vi "Draw Note on Staff.vi"(7 "Landmark C's":bool, 10 "Note Number":i16, 11 "Clef":T1) -> (3 "picture out":picture)   [LabVIEW 2014]
uses:
  Type Defs/Clef.ctl
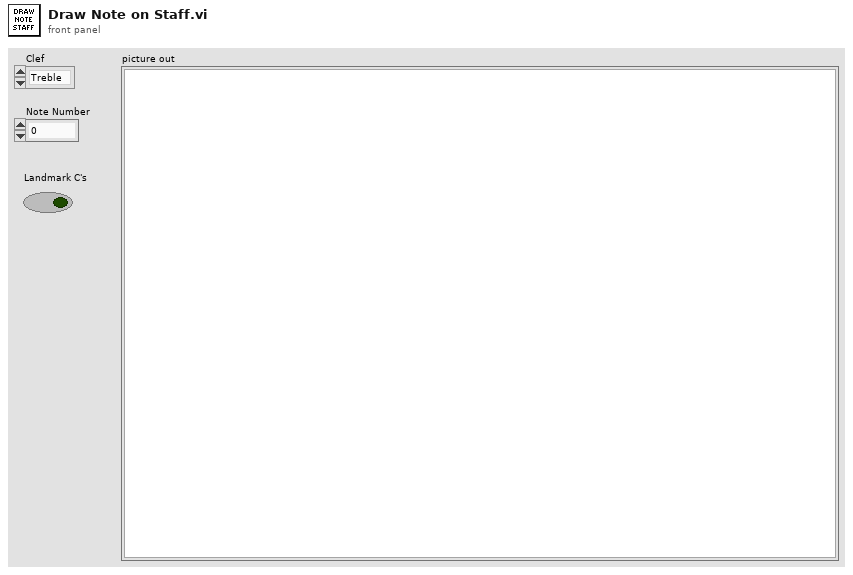
[diagram p1: front panel]
types:
  T1 = typedef "Clef.ctl" = enum16{"Treble", "Bass"}
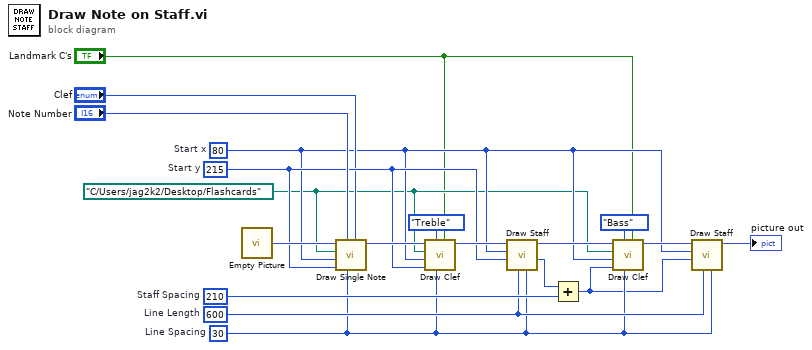
[diagram p0: block diagram]
diagram:
  w2 = path "C:/Users/jag2k2/Desktop/Flashcards" ("Picture Path")
  w12 = i16 215  # Start y
  w7 = i16 80  # Start x
  w19 = i16 210  # Staff Spacing
  w6 = i16 30  # Line Spacing
  w17 = i16 600  # Line Length
  n1 = call "Empty Picture"() -> ("empty picture"=w16:picture)
  n2 = call "Draw Single Note.vi"("Clef"="Clef", "Line Spacing"=w6, "Note Number"="Note Number", "Start y"=w12, "Start x"=w7, "Picture Path"=w2, "Picture In"=w16) -> ("Picture Out"=w14:picture)  [unwired: 4 in]
  n3 = call "Draw Clef.vi"("Landmark C's"="Landmark C's", "Line Spacing"=w6, "Clef"=Clef."Treble", "Start y"=w12, "Start x"=w7, "Picture Path"=w2, "Picture In"=w14) -> ("Picture Out"=w13:picture)  [unwired: 4 in]
  n4 = call "Draw Staff.vi"("Line Spacing"=w6, "Line Length"=w17, "Start y"=w12, "Start x"=w7, "picture in"=w13) -> ("End y"=w18:i16, "picture out"=w9:picture)  [unwired: 5 in]
  n5 = Add(x=w18, y=w19) -> (x+y=w5:i16)
  n6 = call "Draw Clef.vi"("Landmark C's"="Landmark C's", "Line Spacing"=w6, "Clef"=Clef."Bass", "Start y"=w5, "Start x"=w7, "Picture Path"=w2, "Picture In"=w9) -> ("Picture Out"=w8:picture)  [unwired: 4 in]
  n7 = call "Draw Staff.vi"("Line Spacing"=w6, "Line Length"=w17, "Start y"=w5, "Start x"=w7, "picture in"=w8) -> ("picture out"=→"picture out":picture)  [unwired: 5 in, 1 out]
